vi "集成干预.vi"(11 "数据标记表":string(combo)="N") -> ()   [LabVIEW 2016, in "斯坦道多参数.lvlib"]
panel:
  out "运行状态":u16(ring) items=["空闲", "水样测试", "标样核查"]
  out "多参数运行日志":string
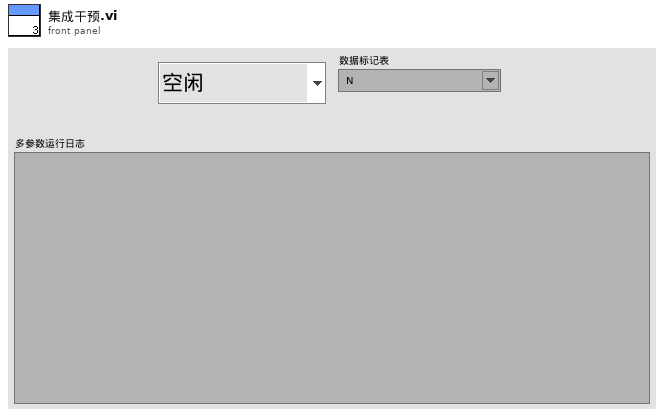
[diagram p1: front panel]
types:
  T1 = typedef "集成多参数单参数字段定义.ctl" = cluster{"时间":timestamp, "测量模式":string, "数据类型":string, "检测值":sgl, "单位":string, "数据标识":string, "信号值":sgl, "标样参考值":sgl, "因子编码":string, "探头温度":sgl, "LastTime":timestamp}
  T2 = cluster{"水温":bool, "pH":bool, "DO":bool, "DOper":bool, "电导率":bool, "ORP":bool, "浊度":bool, "叶绿素a":bool, "藻密度":bool, "COD":bool, "DO2":bool, "DOper":bool, "氯化物":bool, "氨氮":bool, "水中油":bool, "悬浮物":bool, "余氯":bool}
  T3 = cluster{"ph":bool, "DO":bool, "Cond":bool, "Turb":bool, "叶绿素a":bool, "藻密度":bool, "ORP":bool, "cod":bool, "DO2":bool, "氯化物":bool, "氨氮":bool, "水中油":bool, "悬浮物":bool, "余氯":bool}
  T4 = cluster{"温度测量值":sgl, "测量值":sgl, "温度偏移修正值":sgl, "信号值":sgl, "数据标识":string}
  T5 = cluster{"温度测量值":sgl, "DO%":sgl, "DOmg/L":sgl, "温度偏移修正值":sgl, "数据标识mg/L":string, "数据标识%":string}
  T6 = cluster{"CH":u16, "监测值":dbl, "信号值":sgl, "数据标识":string}
  T7 = cluster{"水样数据时间":timestamp, "水温":dbl, "pH":dbl, "DO":dbl, "DOper":dbl, "电导率":dbl, "ORP":dbl, "浊度":dbl, "叶绿素a":dbl, "藻密度":dbl, "COD":dbl, "DO2":dbl, "DO2per":dbl, "氯化物":dbl, "氨氮":dbl, "水中油":dbl, "悬浮物":dbl, "余氯":dbl}
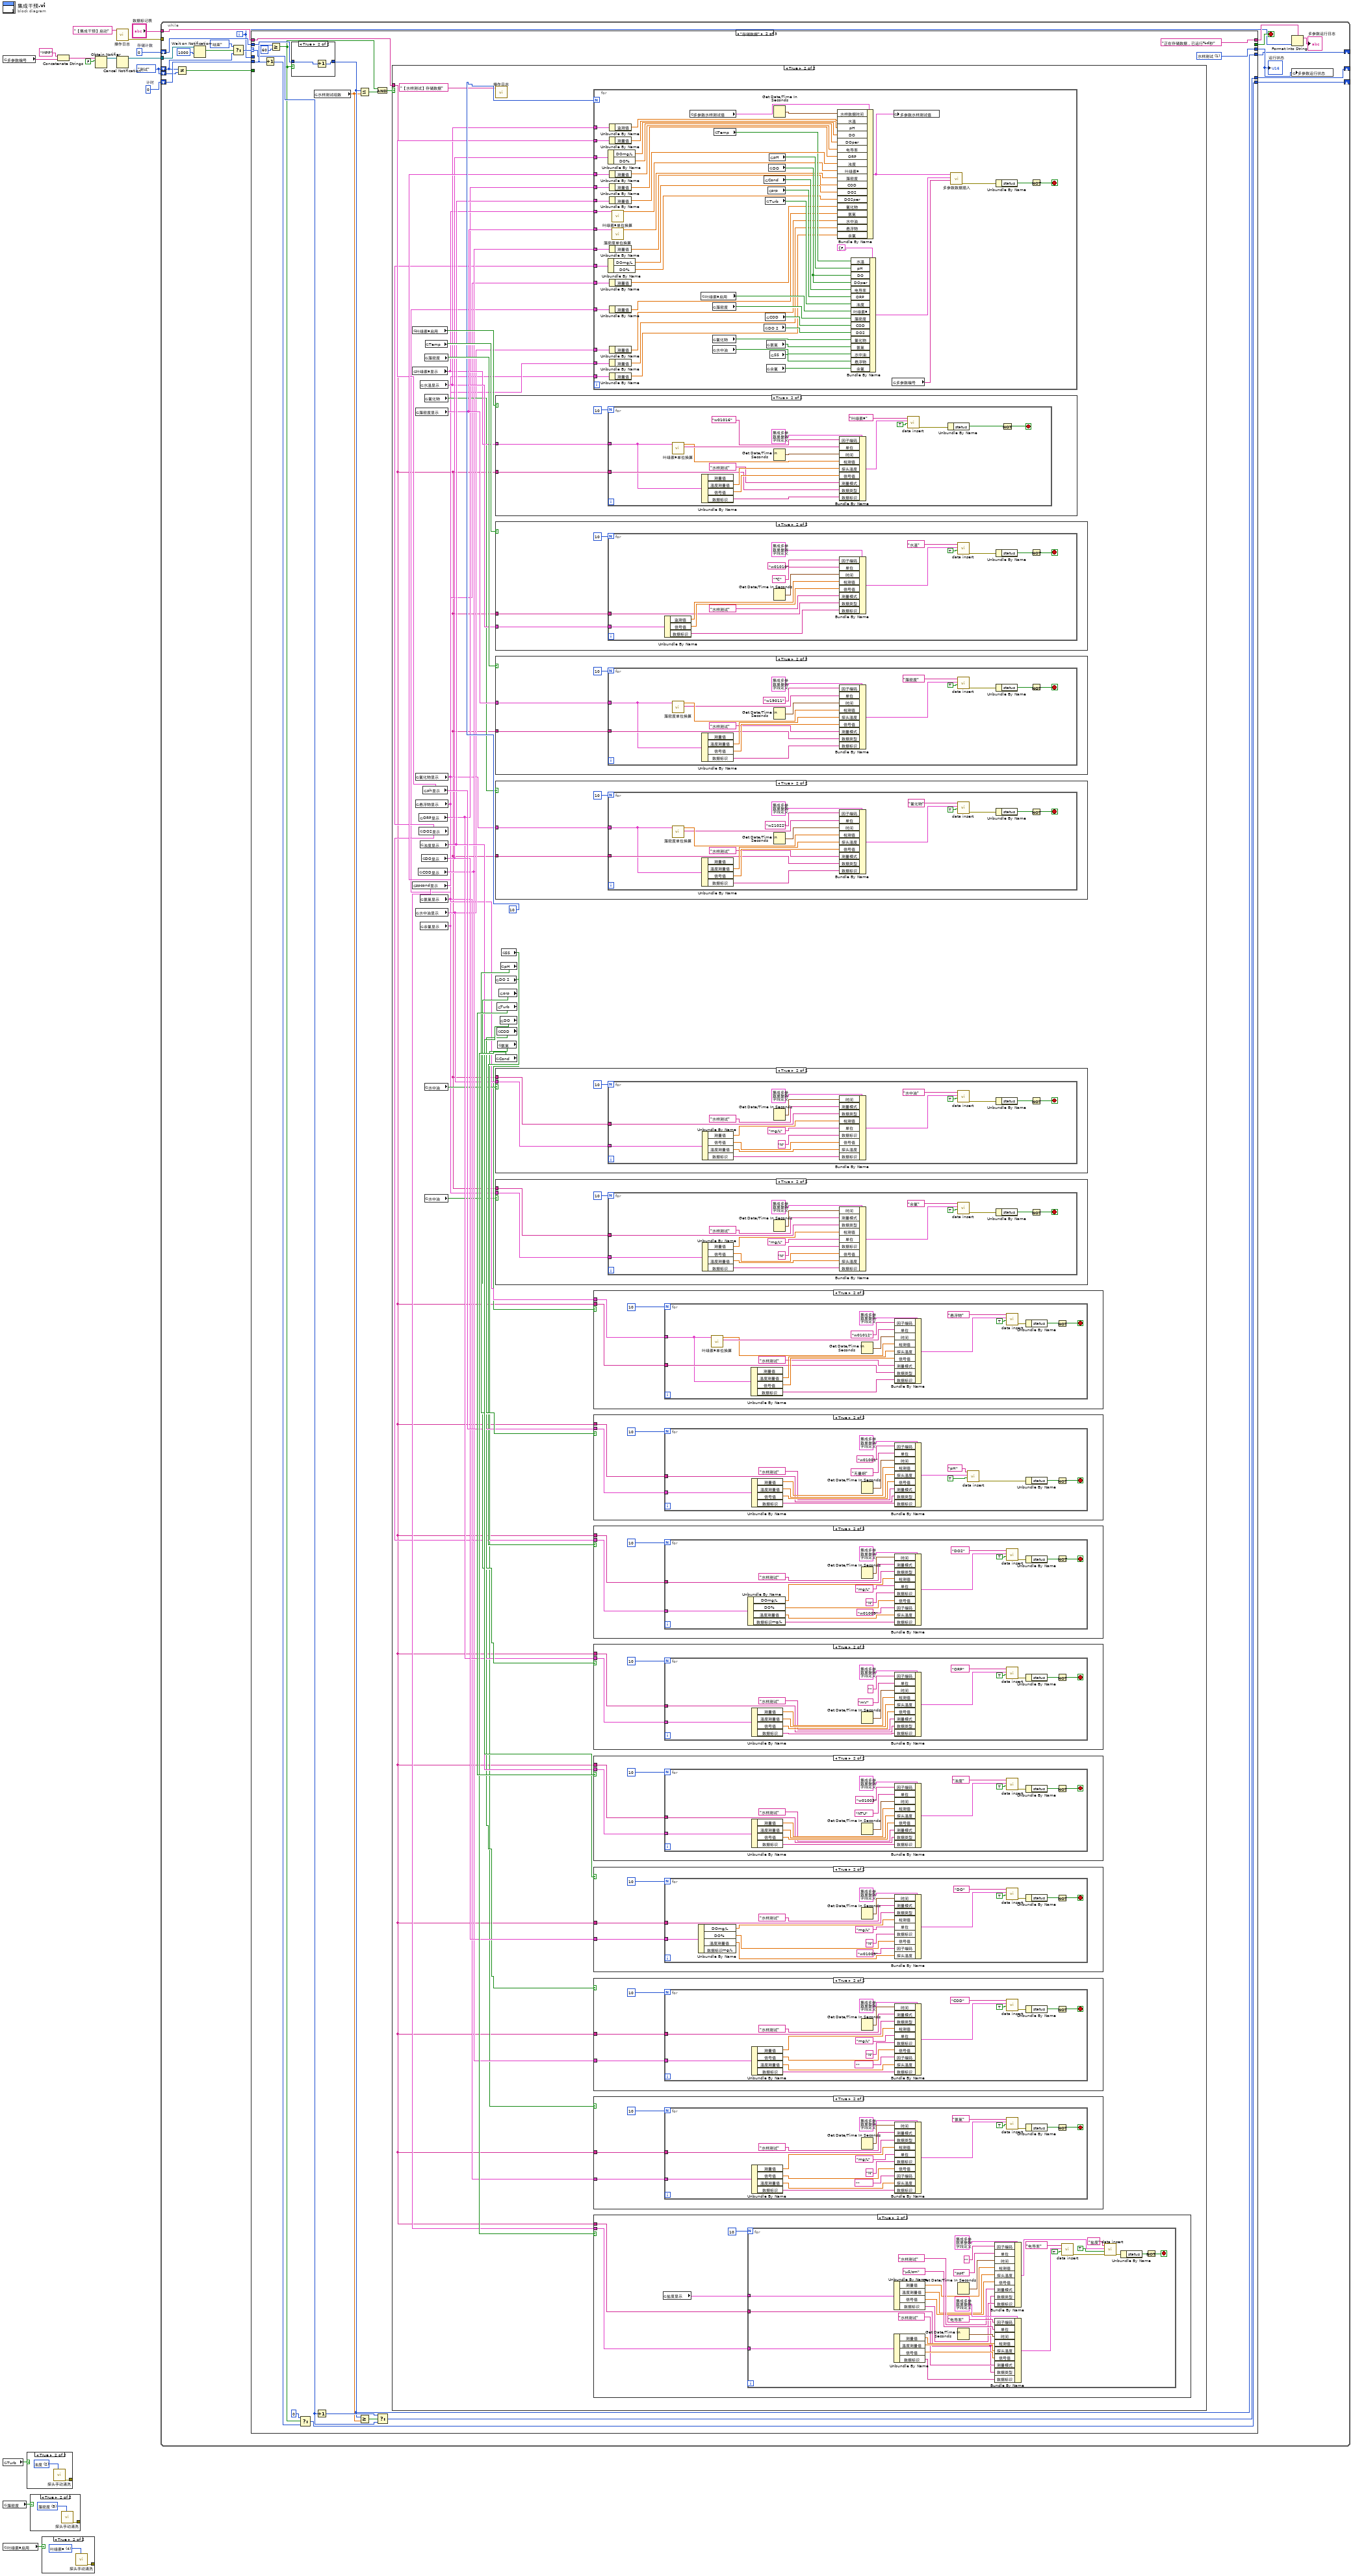
[diagram p0: block diagram]
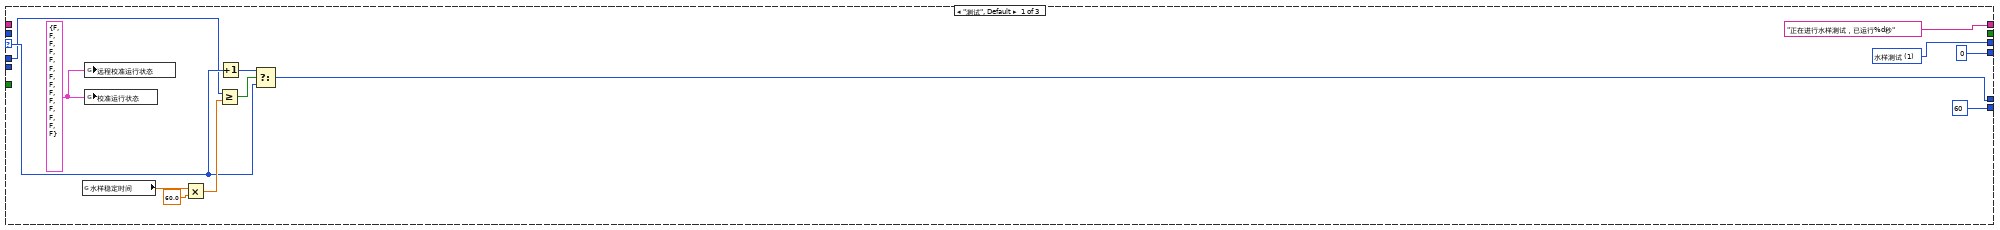
[diagram p5: hidden frame]
diagram:
  w7 = 0  # 存储计数
  w8 = 0  # 计时
  w3 = enum16{"测试", "存储数据", "结束"}."测试" ("枚举")
  n1 = global read "多参数全局变量.vi" "多参数编号"() -> (w9:string)
  n2 = global read "断电保存变量.vi" "Turb"() -> (w6:bool)
  n3 = global read "断电保存变量.vi" "藻密度"() -> (w4:bool)
  n4 = global read "断电保存变量.vi" "叶绿素a启用"() -> (w5:bool)
  n5 = case shown="True" w6 {
    tunnel: [_ w16] -> _
    frame False {
    }
    frame True {
      w17 = u16 2 items=["pH", "DO", "浊度", "电导率", "叶绿素a", "藻密度", "ORP", "DO2"] ("校准参数")
      n6 = call "探头手动清洗.vi"("校准参数"=w17) -> ("error out"=w16:errorcluster)  [unwired: 10 in]
    }
  }
  n7 = case shown="True" w4 {
    tunnel: [_ w18] -> _
    frame False {
    }
    frame True {
      w19 = u16 5 items=["pH", "DO", "浊度", "电导率", "叶绿素a", "藻密度", "ORP", "DO2"] ("校准参数")
      n8 = call "探头手动清洗.vi"("校准参数"=w19) -> ("error out"=w18:errorcluster)  [unwired: 10 in]
    }
  }
  n9 = case shown="True" w5 {
    tunnel: [_ w20] -> _
    frame False {
    }
    frame True {
      w21 = u16 4 items=["pH", "DO", "浊度", "电导率", "叶绿素a", "藻密度", "ORP", "DO2"] ("校准参数")
      n10 = call "探头手动清洗.vi"("校准参数"=w21) -> ("error out"=w20:errorcluster)  [unwired: 10 in]
    }
  }
  n11 = Concatenate Strings("MPP" ("名称（未命名）"), w9) -> (w10:string)
  n12 = Obtain Notifier(name (unnamed)=w10, notification data type=FALSE) -> (notifier out=w13:refnum<notifier>)  [unwired: 2 in, 2 out]
  n13 = call "操作日志.vi"("日志信息"="【集成干预】启动") -> ("error out"=w1:errorcluster)  [unwired: 10 in]
  n14 = Cancel Notification(0:w13) -> (8:w12:refnum<notifier>)  [unwired: 1 in, 2 out]
  n15 = while {
    shift-right: [w26] -> _
    shift-left: w3 -> [w24]
    tunnel: w12 -> [w37]
    tunnel: "数据标记表" -> [w32]
    shift-right: [w28] -> _
    shift-left: w8 -> [w30]
    shift-right: [w27] -> _
    shift-left: w7 -> [w29]
    shift-left: w3 -> [w23]
    tunnel: w1 -> [_]
    i -> [w25]
    stop <- w40 stop-if-true
    n16 = Not Equal?(x=w24, y=w23) -> (x != y?=w22:bool)
    n17 = Wait on Notification(notifier=w37, timeout in ms (-1)=1000 ("超时毫秒(-1)")) -> (notification=w35:bool)  [unwired: 2 in, 3 out]
    n18 = Select(t=enum16{"测试", "存储数据", "结束"}."结束" ("枚举"), s=w35, f=w24) -> (s? t:f=w33:enum16{"测试", "存储数据", "结束"})
    n19 = case shown="\"存储数据\"" w33 {
      selector: w33 -> [w47 w61 _]
      tunnel: [_ _ TRUE] -> w40
      tunnel: ["正在进行水样测试，已运行%d秒" ("格式字符串") "正在存储数据，已运行%d秒" ("格式字符串") "测试停止，累计运行%d秒" ("格式字符串")] -> w39
      tunnel: [w52 w66 w485] -> w31
      tunnel: w32 -> [_ w71 _]
      tunnel: w30 -> [_ w69 _]
      tunnel: w29 -> [_ w70 _]
      tunnel: [60 w54 0] -> w28
      tunnel: [0 w60 0] -> w27
      tunnel: [w45 w64 enum16{"测试", "存储数据", "结束"}."结束" ("枚举")] -> w26
      tunnel: w25 -> [w42 _ _]
      tunnel: w22 -> [_ _ w481]
      frame "测试", Default {
        w41 = T3 {"ph"=FALSE, "DO"=FALSE, "Cond"=FALSE, "Turb"=FALSE, "叶绿素a"=FALSE, "藻密度"=FALSE, "ORP"=FALSE, "cod"=FALSE, "DO2"=FALSE, "氯化物"=FALSE, "氨氮"=FALSE, "水中油"=FALSE, "悬浮物"=FALSE, "余氯"=FALSE} ("远程校准运行状态")
        w52 = u16 1 items=["空闲", "水样测试", "标样核查"] ("多参数运行状态")
        n20 = global read "断电保存变量.vi" "水样稳定时间"() -> (w51:dbl)
        n21 = global write "多参数全局变量.vi" "远程校准运行状态"(w41) -> ()
        n22 = global write "多参数全局变量.vi" "校准运行状态"(w41) -> ()
        n23 = Multiply(x=w51, y=60.0) -> (x*y=w49:dbl)
        n24 = Greater Or Equal?(x=w42, y=w49) -> (x >= y?=w48:bool)
        n25 = Increment(x=w47) -> (x+1=w46:enum16{"测试", "存储数据", "结束"})
        n26 = Select(t=w46, s=w48, f=w47) -> (s? t:f=w45:enum16{"测试", "存储数据", "结束"})
      }
      frame "存储数据" {
        w66 = u16 1 items=["空闲", "水样测试", "标样核查"] ("多参数运行状态")
        n27 = Increment(x=w69) -> (x+1=w56:i32)
        n28 = Greater Or Equal?(x=w69, y=60) -> (x >= y?=w57:bool)
        n29 = case shown="True" w57 {
          tunnel: w70 -> [w72 w74]
          tunnel: [w72 w73] -> w60
          frame False {
          }
          frame True {
            n30 = Increment(x=w74) -> (x+1=w73:i32)
          }
        }
        n31 = Select(t=0, s=w57, f=w56) -> (s? t:f=w54:i32)
        n32 = global read "断电保存变量.vi" "水样测试组数"() -> (w59:dbl)
        n33 = Increment(x=w61) -> (x+1=w62:enum16{"测试", "存储数据", "结束"})
        n34 = Less Or Equal?(x=w60, y=w59) -> (x <= y?=w65:bool)
        n35 = Greater Or Equal?(x=w60, y=w59) -> (x >= y?=w58:bool)
        n36 = And(x=w57, y=w65) -> (x .and. y?=w63:bool)
        n37 = Select(t=w62, s=w58, f=w61) -> (s? t:f=w64:enum16{"测试", "存储数据", "结束"})
        n38 = case shown="True" w63 {
          tunnel: w71 -> [_ w75]
          frame False {
          }
          frame True {
            n39 = global read "断电保存变量.vi" "叶绿素a启用"() -> (w107:bool)
            n40 = global read "多参数全局变量.vi" "叶绿素a显示"() -> (w92:T4)
            n41 = global read "多参数全局变量.vi" "spcond显示"() -> (w98:T4)
            n42 = global read "多参数全局变量.vi" "藻密度显示"() -> (w94:T4)
            n43 = global read "多参数全局变量.vi" "氯化物显示"() -> (w84:T4)
            n44 = global read "多参数全局变量.vi" "悬浮物显示"() -> (w79:T4)
            n45 = global read "多参数全局变量.vi" "水中油显示"() -> (w80:T4)
            n46 = global read "多参数全局变量.vi" "COD显示"() -> (w89:T4)
            n47 = global read "多参数全局变量.vi" "ORP显示"() -> (w91:T4)
            n48 = global read "多参数全局变量.vi" "DO2显示"() -> (w86:T5)
            n49 = global read "多参数全局变量.vi" "水温显示"() -> (w93:T6)
            n50 = global read "多参数全局变量.vi" "浊度显示"() -> (w96:T4)
            n51 = global read "多参数全局变量.vi" "氨氮显示"() -> (w82:T4)
            n52 = global read "多参数全局变量.vi" "余氯显示"() -> (w76:T4)
            n53 = global read "多参数全局变量.vi" "DO显示"() -> (w95:T5)
            n54 = global read "多参数全局变量.vi" "ph显示"() -> (w97:T4)
            n55 = global read "断电保存变量.vi" "藻密度"() -> (w101:bool)
            n56 = global read "断电保存变量.vi" "氯化物"() -> (w85:bool)
            n57 = global read "断电保存变量.vi" "水中油"() -> (w81:bool)
            n58 = global read "断电保存变量.vi" "水中油"() -> (w77:bool)
            n59 = global read "断电保存变量.vi" "Temp"() -> (w102:bool)
            n60 = call "操作日志.vi"("日志信息"="【水样测试】存储数据") -> ()  [unwired: 10 in, 1 out]
            n61 = case shown="True" w107 {
              tunnel: w75 -> [_ w349]
              tunnel: w92 -> [_ w347]
              frame False {
              }
              frame True {
                n62 = for {
                  N: 10 -> [_]
                  tunnel: w349 -> [w356]
                  tunnel: w347 -> [w353]
                  stop <- w360 stop-if-true
                  n63 = call "叶绿素a单位换算.vi"("叶绿素a显示"=w353) -> ("检测值1.单位"=w352:string, "测量值"=w351:sgl)  [unwired: 8 in, 1 out]
                  n64 = Unbundle By Name(w353) -> ("温度测量值"=w366:sgl, "信号值"=w359:sgl, "数据标识"=w355:string)  [unwired: 1 out]
                  n65 = Get Date/Time In Seconds() -> (seconds since 1Jan1904=w358:timestamp)
                  n66 = Bundle By Name(cluster=T1 {"时间"=timestamp(0 s since 1904-01-01), "测量模式"="水样测试", "数据类型"="N", "检测值"=0.0, "单位"="mg/L", "数据标识"="N", "信号值"=0.0, "标样参考值"=0.0, "因子编码"="", "探头温度"=0.0, "LastTime"=timestamp(0 s since 1904-01-01)} ("data"), "因子编码"="w01016", "单位"=w352, "时间"=w358, "检测值"=w351, "探头温度"=w366, "信号值"=w359, "测量模式"="水样测试", "数据类型"=w356, "数据标识"=w355) -> (w364:T1)
                  n67 = call "data insert.vi"("集成干预"=TRUE, "data"=w364, "table in"="叶绿素a" ("table输入")) -> ("error out"=w362:errorcluster)  [unwired: 8 in]
                  n68 = Unbundle By Name(w362) -> ("status"=w361:bool)
                  n69 = Not(x=w361) -> (.not. x?=w360:bool)
                }
              }
            }
            n70 = case shown="True" w102 {
              tunnel: w75 -> [_ w464]
              tunnel: w93 -> [_ w462]
              frame False {
              }
              frame True {
                n71 = for {
                  N: 10 -> [_]
                  tunnel: w464 -> [w469]
                  tunnel: w462 -> [w468]
                  stop <- w473 stop-if-true
                  n72 = Unbundle By Name(w468) -> ("监测值"=w476:dbl, "信号值"=w471:sgl, "数据标识"=w467:string)
                  n73 = Get Date/Time In Seconds() -> (seconds since 1Jan1904=w472:timestamp)
                  n74 = Bundle By Name(cluster=T1 {"时间"=timestamp(0 s since 1904-01-01), "测量模式"="水样测试", "数据类型"="N", "检测值"=0.0, "单位"="mg/L", "数据标识"="N", "信号值"=0.0, "标样参考值"=0.0, "因子编码"="", "探头温度"=0.0, "LastTime"=timestamp(0 s since 1904-01-01)} ("data"), "因子编码"="w01010", "单位"="℃", "时间"=w472, "检测值"=w476, "信号值"=w471, "测量模式"="水样测试", "数据类型"=w469, "数据标识"=w467) -> (w479:T1)
                  n75 = call "data insert.vi"("集成干预"=TRUE, "data"=w479, "table in"="水温" ("table输入")) -> ("error out"=w475:errorcluster)  [unwired: 8 in]
                  n76 = Unbundle By Name(w475) -> ("status"=w474:bool)
                  n77 = Not(x=w474) -> (.not. x?=w473:bool)
                }
              }
            }
            n78 = case shown="True" w101 {
              tunnel: w75 -> [_ w329]
              tunnel: w94 -> [_ w327]
              frame False {
              }
              frame True {
                n79 = for {
                  N: 10 -> [_]
                  tunnel: w329 -> [w337]
                  tunnel: w327 -> [w333]
                  stop <- w338 stop-if-true
                  n80 = call "藻密度单位换算.vi"("藻密度显示"=w333) -> ("检测值1.单位"=w331:string, "测量值"=w332:sgl)  [unwired: 8 in, 1 out]
                  n81 = Unbundle By Name(w333) -> ("温度测量值"=w346:sgl, "信号值"=w339:sgl, "数据标识"=w335:string)  [unwired: 1 out]
                  n82 = Get Date/Time In Seconds() -> (seconds since 1Jan1904=w340:timestamp)
                  n83 = Bundle By Name(cluster=T1 {"时间"=timestamp(0 s since 1904-01-01), "测量模式"="水样测试", "数据类型"="N", "检测值"=0.0, "单位"="mg/L", "数据标识"="N", "信号值"=0.0, "标样参考值"=0.0, "因子编码"="", "探头温度"=0.0, "LastTime"=timestamp(0 s since 1904-01-01)} ("data"), "因子编码"="w19011", "单位"=w331, "时间"=w340, "检测值"=w332, "探头温度"=w346, "信号值"=w339, "测量模式"="水样测试", "数据类型"=w337, "数据标识"=w335) -> (w341:T1)
                  n84 = call "data insert.vi"("集成干预"=TRUE, "data"=w341, "table in"="藻密度" ("table输入")) -> ("error out"=w343:errorcluster)  [unwired: 8 in]
                  n85 = Unbundle By Name(w343) -> ("status"=w342:bool)
                  n86 = Not(x=w342) -> (.not. x?=w338:bool)
                }
              }
            }
            n87 = case shown="True" w85 {
              tunnel: w75 -> [_ w191]
              tunnel: w84 -> [_ w189]
              frame False {
              }
              frame True {
                n88 = for {
                  N: 10 -> [_]
                  tunnel: w191 -> [w201]
                  tunnel: w189 -> [w197]
                  stop <- w202 stop-if-true
                  n89 = call "藻密度单位换算.vi"("藻密度显示"=w197) -> ("检测值1.单位"=w195:string, "测量值"=w196:sgl)  [unwired: 8 in, 1 out]
                  n90 = Unbundle By Name(w197) -> ("温度测量值"=w208:sgl, "信号值"=w203:sgl, "数据标识"=w199:string)  [unwired: 1 out]
                  n91 = Get Date/Time In Seconds() -> (seconds since 1Jan1904=w204:timestamp)
                  n92 = Bundle By Name(cluster=T1 {"时间"=timestamp(0 s since 1904-01-01), "测量模式"="水样测试", "数据类型"="N", "检测值"=0.0, "单位"="mg/L", "数据标识"="N", "信号值"=0.0, "标样参考值"=0.0, "因子编码"="", "探头温度"=0.0, "LastTime"=timestamp(0 s since 1904-01-01)} ("data"), "因子编码"="w21022", "单位"=w195, "时间"=w204, "检测值"=w196, "探头温度"=w208, "信号值"=w203, "测量模式"="水样测试", "数据类型"=w201, "数据标识"=w199) -> (w205:T1)
                  n93 = call "data insert.vi"("集成干预"=TRUE, "data"=w205, "table in"="氯化物") -> ("error out"=w207:errorcluster)  [unwired: 8 in]
                  n94 = Unbundle By Name(w207) -> ("status"=w206:bool)
                  n95 = Not(x=w206) -> (.not. x?=w202:bool)
                }
              }
            }
            n96 = global read "断电保存变量.vi" "DO 2"() -> (w87:bool)
            n97 = global read "断电保存变量.vi" "Cond"() -> (w105:bool)
            n98 = case shown="True" w81 {
              tunnel: w75 -> [_ w150]
              tunnel: w80 -> [_ w148]
              frame False {
              }
              frame True {
                n99 = for {
                  N: 10 -> [_]
                  tunnel: w150 -> [w164]
                  tunnel: w148 -> [w157]
                  stop <- w167 stop-if-true
                  n100 = Unbundle By Name(w157) -> ("测量值"=w156:sgl, "信号值"=w155:sgl, "温度测量值"=w154:sgl, "数据标识"=w153:string)
                  n101 = Get Date/Time In Seconds() -> (seconds since 1Jan1904=w166:timestamp)
                  n102 = Bundle By Name(cluster=T1 {"时间"=timestamp(0 s since 1904-01-01), "测量模式"="水样测试", "数据类型"="N", "检测值"=0.0, "单位"="mg/L", "数据标识"="N", "信号值"=0.0, "标样参考值"=0.0, "因子编码"="", "探头温度"=0.0, "LastTime"=timestamp(0 s since 1904-01-01)} ("data"), "时间"=w166, "测量模式"="水样测试", "数据类型"=w164, "检测值"=w156, "单位"="mg/L", "数据标识"="N" ("水样数据标识"), "信号值"=w155, "探头温度"=w154, "数据标识"=w153) -> (w159:T1)
                  n103 = call "data insert.vi"("集成干预"=TRUE, "data"=w159, "table in"="水中油") -> ("error out"=w160:errorcluster)  [unwired: 8 in]
                  n104 = Unbundle By Name(w160) -> ("status"=w161:bool)
                  n105 = Not(x=w161) -> (.not. x?=w167:bool)
                }
              }
            }
            n106 = case shown="True" w77 {
              tunnel: w75 -> [_ w110]
              tunnel: w76 -> [_ w108]
              frame False {
              }
              frame True {
                n107 = for {
                  N: 10 -> [_]
                  tunnel: w110 -> [w124]
                  tunnel: w108 -> [w117]
                  stop <- w127 stop-if-true
                  n108 = Unbundle By Name(w117) -> ("测量值"=w116:sgl, "信号值"=w115:sgl, "温度测量值"=w114:sgl, "数据标识"=w113:string)
                  n109 = Get Date/Time In Seconds() -> (seconds since 1Jan1904=w126:timestamp)
                  n110 = Bundle By Name(cluster=T1 {"时间"=timestamp(0 s since 1904-01-01), "测量模式"="水样测试", "数据类型"="N", "检测值"=0.0, "单位"="mg/L", "数据标识"="N", "信号值"=0.0, "标样参考值"=0.0, "因子编码"="", "探头温度"=0.0, "LastTime"=timestamp(0 s since 1904-01-01)} ("data"), "时间"=w126, "测量模式"="水样测试", "数据类型"=w124, "检测值"=w116, "单位"="mg/L", "数据标识"="N" ("水样数据标识"), "信号值"=w115, "探头温度"=w114, "数据标识"=w113) -> (w119:T1)
                  n111 = call "data insert.vi"("集成干预"=TRUE, "data"=w119, "table in"="余氯") -> ("error out"=w120:errorcluster)  [unwired: 8 in]
                  n112 = Unbundle By Name(w120) -> ("status"=w121:bool)
                  n113 = Not(x=w121) -> (.not. x?=w127:bool)
                }
              }
            }
            n114 = global read "断电保存变量.vi" "Turb"() -> (w106:bool)
            n115 = global read "断电保存变量.vi" "COD"() -> (w88:bool)
            n116 = global read "断电保存变量.vi" "氨氮"() -> (w83:bool)
            n117 = global read "断电保存变量.vi" "orp"() -> (w100:bool)
            n118 = global read "断电保存变量.vi" "DO"() -> (w104:bool)
            n119 = global read "断电保存变量.vi" "pH"() -> (w103:bool)
            n120 = global read "断电保存变量.vi" "SS"() -> (w78:bool)
            n121 = for {
              N: 10 -> [_]
              tunnel: w93 -> [w286]
              tunnel: w97 -> [w285]
              tunnel: w95 -> [w284]
              tunnel: w98 -> [w283]
              tunnel: w91 -> [w282]
              tunnel: w96 -> [w281]
              tunnel: w92 -> [w271]
              tunnel: w94 -> [w273]
              tunnel: w89 -> [w279]
              tunnel: w86 -> [w276]
              tunnel: w84 -> [w267]
              tunnel: w82 -> [w265]
              tunnel: w80 -> [w260]
              tunnel: w79 -> [w254]
              tunnel: w76 -> [w252]
              stop <- w288 stop-if-true
              n122 = Unbundle By Name(w284) -> ("DOmg/L"=w303:sgl, "DO%"=w302:sgl)
              n123 = Unbundle By Name(w276) -> ("DOmg/L"=w275:sgl, "DO%"=w274:sgl)
              n124 = Unbundle By Name(w286) -> ("监测值"=w305:dbl)
              n125 = Unbundle By Name(w285) -> ("测量值"=w304:sgl)
              n126 = Unbundle By Name(w283) -> ("测量值"=w301:sgl)
              n127 = Unbundle By Name(w282) -> ("测量值"=w300:sgl)
              n128 = Unbundle By Name(w281) -> ("测量值"=w299:sgl)
              n129 = Unbundle By Name(w279) -> ("测量值"=w278:sgl)
              n130 = Unbundle By Name(w267) -> ("测量值"=w266:sgl)
              n131 = Unbundle By Name(w265) -> ("测量值"=w264:sgl)
              n132 = Unbundle By Name(w260) -> ("测量值"=w259:sgl)
              n133 = Unbundle By Name(w254) -> ("测量值"=w255:sgl)
              n134 = Unbundle By Name(w252) -> ("测量值"=w251:sgl)
              n135 = call "叶绿素a单位换算.vi"("叶绿素a显示"=w271) -> ("测量值"=w270:sgl)  [unwired: 8 in, 2 out]
              n136 = call "藻密度单位换算.vi"("藻密度显示"=w273) -> ("测量值"=w272:sgl)  [unwired: 8 in, 2 out]
              n137 = global read "多参数全局变量.vi" "多参数水样测试值"() -> (w262:T7)
              n138 = global read "断电保存变量.vi" "叶绿素a启用"() -> (w292:bool)
              n139 = global read "断电保存变量.vi" "藻密度"() -> (w295:bool)
              n140 = global read "断电保存变量.vi" "氯化物"() -> (w268:bool)
              n141 = global read "断电保存变量.vi" "水中油"() -> (w261:bool)
              n142 = global read "断电保存变量.vi" "Temp"() -> (w294:bool)
              n143 = global read "断电保存变量.vi" "Cond"() -> (w297:bool)
              n144 = global read "断电保存变量.vi" "DO 2"() -> (w277:bool)
              n145 = global read "断电保存变量.vi" "Turb"() -> (w296:bool)
              n146 = global read "断电保存变量.vi" "COD"() -> (w280:bool)
              n147 = global read "断电保存变量.vi" "氨氮"() -> (w263:bool)
              n148 = global read "断电保存变量.vi" "余氯"() -> (w253:bool)
              n149 = global read "断电保存变量.vi" "orp"() -> (w293:bool)
              n150 = global read "断电保存变量.vi" "DO"() -> (w291:bool)
              n151 = global read "断电保存变量.vi" "pH"() -> (w298:bool)
              n152 = global read "断电保存变量.vi" "SS"() -> (w258:bool)
              n153 = Get Date/Time In Seconds() -> (seconds since 1Jan1904=w306:timestamp)
              n154 = Bundle By Name(cluster=w262, "水样数据时间"=w306, "水温"=w305, "pH"=w304, "DO"=w303, "DOper"=w302, "电导率"=w301, "ORP"=w300, "浊度"=w299, "叶绿素a"=w270, "藻密度"=w272, "COD"=w278, "DO2"=w275, "DO2per"=w274, "氯化物"=w266, "氨氮"=w264, "水中油"=w259, "悬浮物"=w255, "余氯"=w251) -> (w269:T7)
              n155 = Bundle By Name(cluster=T2 {"水温"=FALSE, "pH"=FALSE, "DO"=FALSE, "DOper"=FALSE, "电导率"=FALSE, "ORP"=FALSE, "浊度"=FALSE, "叶绿素a"=FALSE, "藻密度"=FALSE, "COD"=FALSE, "DO2"=FALSE, "DOper"=FALSE, "氯化物"=FALSE, "氨氮"=FALSE, "水中油"=FALSE, "悬浮物"=FALSE, "余氯"=FALSE} ("columns enable"), "水温"=w294, "pH"=w298, "DO"=w291, "DOper"=w291, "电导率"=w297, "ORP"=w293, "浊度"=w296, "叶绿素a"=w292, "藻密度"=w295, "COD"=w280, "DO2"=w277, "氯化物"=w268, "氨氮"=w263, "水中油"=w261, "悬浮物"=w258, "余氯"=w253) -> (w256:T2)
              n156 = global read "多参数全局变量.vi" "多参数编号"() -> (w287:string)
              n157 = global write "多参数全局变量.vi" "多参数水样测试值"(w269) -> ()
              n158 = call "多参数数据插入.vi"("编号"=w287, "columns enable"=w256, "data in"=w269) -> ("error out"=w290:errorcluster)  [unwired: 8 in]
              n159 = Unbundle By Name(w290) -> ("status"=w289:bool)
              n160 = Not(x=w289) -> (.not. x?=w288:bool)
            }
            n161 = case shown="True" w78 {
              tunnel: w75 -> [_ w130]
              tunnel: w79 -> [_ w128]
              frame False {
              }
              frame True {
                n162 = for {
                  N: 10 -> [_]
                  tunnel: w130 -> [w137]
                  tunnel: w128 -> [w134]
                  stop <- w141 stop-if-true
                  n163 = call "叶绿素a单位换算.vi"("叶绿素a显示"=w134) -> ("检测值1.单位"=w133:string, "测量值"=w132:sgl)  [unwired: 8 in, 1 out]
                  n164 = Unbundle By Name(w134) -> ("温度测量值"=w147:sgl, "信号值"=w140:sgl, "数据标识"=w136:string)  [unwired: 1 out]
                  n165 = Get Date/Time In Seconds() -> (seconds since 1Jan1904=w139:timestamp)
                  n166 = Bundle By Name(cluster=T1 {"时间"=timestamp(0 s since 1904-01-01), "测量模式"="水样测试", "数据类型"="N", "检测值"=0.0, "单位"="mg/L", "数据标识"="N", "信号值"=0.0, "标样参考值"=0.0, "因子编码"="", "探头温度"=0.0, "LastTime"=timestamp(0 s since 1904-01-01)} ("data"), "因子编码"="w01012", "单位"=w133, "时间"=w139, "检测值"=w132, "探头温度"=w147, "信号值"=w140, "测量模式"="水样测试", "数据类型"=w137, "数据标识"=w136) -> (w145:T1)
                  n167 = call "data insert.vi"("集成干预"=TRUE, "data"=w145, "table in"="悬浮物" ("table输入")) -> ("error out"=w143:errorcluster)  [unwired: 8 in]
                  n168 = Unbundle By Name(w143) -> ("status"=w142:bool)
                  n169 = Not(x=w142) -> (.not. x?=w141:bool)
                }
              }
            }
            n170 = case shown="True" w103 {
              tunnel: w75 -> [_ w444]
              tunnel: w97 -> [_ w442]
              frame False {
              }
              frame True {
                n171 = for {
                  N: 10 -> [_]
                  tunnel: w444 -> [w449]
                  tunnel: w442 -> [w448]
                  stop <- w453 stop-if-true
                  n172 = Unbundle By Name(w448) -> ("测量值"=w457:sgl, "温度测量值"=w456:sgl, "信号值"=w451:sgl, "数据标识"=w447:string)
                  n173 = Get Date/Time In Seconds() -> (seconds since 1Jan1904=w452:timestamp)
                  n174 = Bundle By Name(cluster=T1 {"时间"=timestamp(0 s since 1904-01-01), "测量模式"="水样测试", "数据类型"="N", "检测值"=0.0, "单位"="mg/L", "数据标识"="N", "信号值"=0.0, "标样参考值"=0.0, "因子编码"="", "探头温度"=0.0, "LastTime"=timestamp(0 s since 1904-01-01)} ("data"), "因子编码"="w01001", "单位"="无量纲", "时间"=w452, "检测值"=w457, "探头温度"=w456, "信号值"=w451, "测量模式"="水样测试", "数据类型"=w449, "数据标识"=w447) -> (w461:T1)
                  n175 = call "data insert.vi"("集成干预"=TRUE, "data"=w461, "table in"="pH" ("table输入")) -> ("error out"=w455:errorcluster)  [unwired: 8 in]
                  n176 = Unbundle By Name(w455) -> ("status"=w454:bool)
                  n177 = Not(x=w454) -> (.not. x?=w453:bool)
                }
              }
            }
            n178 = case shown="True" w87 {
              tunnel: w75 -> [_ w211]
              tunnel: w86 -> [_ w209]
              frame False {
              }
              frame True {
                n179 = for {
                  N: 10 -> [_]
                  tunnel: w211 -> [w226]
                  tunnel: w209 -> [w216]
                  stop <- w229 stop-if-true
                  n180 = Unbundle By Name(w216) -> ("DOmg/L"=w225:sgl, "DO%"=w218:sgl, "温度测量值"=w219:sgl, "数据标识mg/L"=w215:string)
                  n181 = Get Date/Time In Seconds() -> (seconds since 1Jan1904=w228:timestamp)
                  n182 = Bundle By Name(cluster=T1 {"时间"=timestamp(0 s since 1904-01-01), "测量模式"="水样测试", "数据类型"="N", "检测值"=0.0, "单位"="mg/L", "数据标识"="N", "信号值"=0.0, "标样参考值"=0.0, "因子编码"="", "探头温度"=0.0, "LastTime"=timestamp(0 s since 1904-01-01)} ("data"), "时间"=w228, "测量模式"="水样测试", "数据类型"=w226, "检测值"=w225, "单位"="mg/L", "数据标识"="N" ("水样数据标识"), "信号值"=w218, "因子编码"="w01009", "探头温度"=w219, "数据标识"=w215) -> (w217:T1)
                  n183 = call "data insert.vi"("集成干预"=TRUE, "data"=w217, "table in"="DO2") -> ("error out"=w221:errorcluster)  [unwired: 8 in]
                  n184 = Unbundle By Name(w221) -> ("status"=w222:bool)
                  n185 = Not(x=w222) -> (.not. x?=w229:bool)
                }
              }
            }
            n186 = case shown="True" w100 {
              tunnel: w75 -> [_ w309]
              tunnel: w91 -> [_ w307]
              frame False {
              }
              frame True {
                n187 = for {
                  N: 10 -> [_]
                  tunnel: w309 -> [w316]
                  tunnel: w307 -> [w314]
                  stop <- w319 stop-if-true
                  n188 = Unbundle By Name(w314) -> ("测量值"=w326:sgl, "温度测量值"=w324:sgl, "信号值"=w317:sgl, "数据标识"=w313:string)
                  n189 = Get Date/Time In Seconds() -> (seconds since 1Jan1904=w318:timestamp)
                  n190 = Bundle By Name(cluster=T1 {"时间"=timestamp(0 s since 1904-01-01), "测量模式"="水样测试", "数据类型"="N", "检测值"=0.0, "单位"="mg/L", "数据标识"="N", "信号值"=0.0, "标样参考值"=0.0, "因子编码"="", "探头温度"=0.0, "LastTime"=timestamp(0 s since 1904-01-01)} ("data"), "因子编码"="", "单位"="mV", "时间"=w318, "检测值"=w326, "探头温度"=w324, "信号值"=w317, "测量模式"="水样测试", "数据类型"=w316, "数据标识"=w313) -> (w311:T1)
                  n191 = call "data insert.vi"("集成干预"=TRUE, "data"=w311, "table in"="ORP" ("table输入")) -> ("error out"=w322:errorcluster)  [unwired: 8 in]
                  n192 = Unbundle By Name(w322) -> ("status"=w321:bool)
                  n193 = Not(x=w321) -> (.not. x?=w319:bool)
                }
              }
            }
            n194 = case shown="True" w106 {
              tunnel: w75 -> [_ w369]
              tunnel: w96 -> [_ w367]
              frame False {
              }
              frame True {
                n195 = for {
                  N: 10 -> [_]
                  tunnel: w369 -> [w374]
                  tunnel: w367 -> [w373]
                  stop <- w378 stop-if-true
                  n196 = Unbundle By Name(w373) -> ("测量值"=w382:sgl, "温度测量值"=w381:sgl, "信号值"=w376:sgl, "数据标识"=w372:string)
                  n197 = Get Date/Time In Seconds() -> (seconds since 1Jan1904=w377:timestamp)
                  n198 = Bundle By Name(cluster=T1 {"时间"=timestamp(0 s since 1904-01-01), "测量模式"="水样测试", "数据类型"="N", "检测值"=0.0, "单位"="mg/L", "数据标识"="N", "信号值"=0.0, "标样参考值"=0.0, "因子编码"="", "探头温度"=0.0, "LastTime"=timestamp(0 s since 1904-01-01)} ("data"), "因子编码"="w01003", "单位"="NTU", "时间"=w377, "检测值"=w382, "探头温度"=w381, "信号值"=w376, "测量模式"="水样测试", "数据类型"=w374, "数据标识"=w372) -> (w385:T1)
                  n199 = call "data insert.vi"("集成干预"=TRUE, "data"=w385, "table in"="浊度" ("table输入")) -> ("error out"=w380:errorcluster)  [unwired: 8 in]
                  n200 = Unbundle By Name(w380) -> ("status"=w379:bool)
                  n201 = Not(x=w379) -> (.not. x?=w378:bool)
                }
              }
            }
            n202 = case shown="True" w104 {
              tunnel: w75 -> [_ w424]
              tunnel: w95 -> [_ w422]
              frame False {
              }
              frame True {
                n203 = for {
                  N: 10 -> [_]
                  tunnel: w424 -> [w437]
                  tunnel: w422 -> [w428]
                  stop <- w441 stop-if-true
                  n204 = Unbundle By Name(w428) -> ("DOmg/L"=w436:sgl, "DO%"=w430:sgl, "温度测量值"=w431:sgl)  [unwired: 1 out]
                  n205 = Get Date/Time In Seconds() -> (seconds since 1Jan1904=w439:timestamp)
                  n206 = Bundle By Name(cluster=T1 {"时间"=timestamp(0 s since 1904-01-01), "测量模式"="水样测试", "数据类型"="N", "检测值"=0.0, "单位"="mg/L", "数据标识"="N", "信号值"=0.0, "标样参考值"=0.0, "因子编码"="", "探头温度"=0.0, "LastTime"=timestamp(0 s since 1904-01-01)} ("data"), "时间"=w439, "测量模式"="水样测试", "数据类型"=w437, "检测值"=w436, "单位"="mg/L", "数据标识"="N", "信号值"=w430, "因子编码"="w01009", "探头温度"=w431) -> (w429:T1)
                  n207 = call "data insert.vi"("集成干预"=TRUE, "data"=w429, "table in"="DO") -> ("error out"=w433:errorcluster)  [unwired: 8 in]
                  n208 = Unbundle By Name(w433) -> ("status"=w434:bool)
                  n209 = Not(x=w434) -> (.not. x?=w441:bool)
                }
              }
            }
            n210 = case shown="True" w88 {
              tunnel: w75 -> [_ w232]
              tunnel: w89 -> [_ w230]
              frame False {
              }
              frame True {
                n211 = for {
                  N: 10 -> [_]
                  tunnel: w232 -> [w246]
                  tunnel: w230 -> [w236]
                  stop <- w250 stop-if-true
                  n212 = Unbundle By Name(w236) -> ("测量值"=w245:sgl, "信号值"=w238:sgl, "温度测量值"=w239:sgl, "数据标识"=w235:string)
                  n213 = Get Date/Time In Seconds() -> (seconds since 1Jan1904=w248:timestamp)
                  n214 = Bundle By Name(cluster=T1 {"时间"=timestamp(0 s since 1904-01-01), "测量模式"="水样测试", "数据类型"="N", "检测值"=0.0, "单位"="mg/L", "数据标识"="N", "信号值"=0.0, "标样参考值"=0.0, "因子编码"="", "探头温度"=0.0, "LastTime"=timestamp(0 s since 1904-01-01)} ("data"), "时间"=w248, "测量模式"="水样测试", "数据类型"=w246, "检测值"=w245, "单位"="mg/L", "数据标识"="N" ("水样数据标识"), "信号值"=w238, "因子编码"="", "探头温度"=w239, "数据标识"=w235) -> (w237:T1)
                  n215 = call "data insert.vi"("集成干预"=TRUE, "data"=w237, "table in"="COD") -> ("error out"=w241:errorcluster)  [unwired: 8 in]
                  n216 = Unbundle By Name(w241) -> ("status"=w242:bool)
                  n217 = Not(x=w242) -> (.not. x?=w250:bool)
                }
              }
            }
            n218 = case shown="True" w83 {
              tunnel: w75 -> [_ w170]
              tunnel: w82 -> [_ w168]
              frame False {
              }
              frame True {
                n219 = for {
                  N: 10 -> [_]
                  tunnel: w170 -> [w184]
                  tunnel: w168 -> [w176]
                  stop <- w188 stop-if-true
                  n220 = Unbundle By Name(w176) -> ("测量值"=w175:sgl, "信号值"=w174:sgl, "温度测量值"=w173:sgl, "数据标识"=w172:string)
                  n221 = Get Date/Time In Seconds() -> (seconds since 1Jan1904=w186:timestamp)
                  n222 = Bundle By Name(cluster=T1 {"时间"=timestamp(0 s since 1904-01-01), "测量模式"="水样测试", "数据类型"="N", "检测值"=0.0, "单位"="mg/L", "数据标识"="N", "信号值"=0.0, "标样参考值"=0.0, "因子编码"="", "探头温度"=0.0, "LastTime"=timestamp(0 s since 1904-01-01)} ("data"), "时间"=w186, "测量模式"="水样测试", "数据类型"=w184, "检测值"=w175, "单位"="mg/L", "数据标识"="N" ("水样数据标识"), "信号值"=w174, "因子编码"="", "探头温度"=w173, "数据标识"=w172) -> (w178:T1)
                  n223 = call "data insert.vi"("集成干预"=TRUE, "data"=w178, "table in"="氨氮") -> ("error out"=w180:errorcluster)  [unwired: 8 in]
                  n224 = Unbundle By Name(w180) -> ("status"=w181:bool)
                  n225 = Not(x=w181) -> (.not. x?=w188:bool)
                }
              }
            }
            n226 = case shown="True" w105 {
              tunnel: w75 -> [_ w390]
              tunnel: w98 -> [_ w388]
              frame False {
              }
              frame True {
                n227 = global read "多参数全局变量.vi" "盐度显示"() -> (w387:T4)
                n228 = for {
                  N: 10 -> [_]
                  tunnel: w390 -> [w398]
                  tunnel: w388 -> [w410]
                  tunnel: w387 -> [w397]
                  stop <- w415 stop-if-true
                  n229 = Unbundle By Name(w397) -> ("测量值"=w399:sgl, "温度测量值"=w400:sgl, "信号值"=w403:sgl, "数据标识"=w406:string)
                  n230 = Unbundle By Name(w410) -> ("测量值"=w419:sgl, "温度测量值"=w418:sgl, "信号值"=w413:sgl, "数据标识"=w409:string)
                  n231 = Get Date/Time In Seconds() -> (seconds since 1Jan1904=w402:timestamp)
                  n232 = Get Date/Time In Seconds() -> (seconds since 1Jan1904=w414:timestamp)
                  n233 = Bundle By Name(cluster=T1 {"时间"=timestamp(0 s since 1904-01-01), "测量模式"="水样测试", "数据类型"="N", "检测值"=0.0, "单位"="mg/L", "数据标识"="N", "信号值"=0.0, "标样参考值"=0.0, "因子编码"="", "探头温度"=0.0, "LastTime"=timestamp(0 s since 1904-01-01)} ("data"), "因子编码"="", "单位"="ppt", "时间"=w402, "检测值"=w399, "探头温度"=w400, "信号值"=w403, "测量模式"="水样测试", "数据类型"=w398, "数据标识"=w406) -> (w405:T1)
                  n234 = Bundle By Name(cluster=T1 {"时间"=timestamp(0 s since 1904-01-01), "测量模式"="水样测试", "数据类型"="N", "检测值"=0.0, "单位"="mg/L", "数据标识"="N", "信号值"=0.0, "标样参考值"=0.0, "因子编码"="", "探头温度"=0.0, "LastTime"=timestamp(0 s since 1904-01-01)} ("data"), "因子编码"="电导率", "单位"="μS/cm", "时间"=w414, "检测值"=w419, "探头温度"=w418, "信号值"=w413, "测量模式"="水样测试", "数据类型"=w398, "数据标识"=w409) -> (w411:T1)
                  n235 = call "data insert.vi"("集成干预"=TRUE, "data"=w411, "table in"="电导率" ("table输入")) -> ("error out"=w394:errorcluster)  [unwired: 8 in]
                  n236 = call "data insert.vi"("error in (no error)"=w394, "集成干预"=TRUE, "data"=w405, "table in"="盐度") -> ("error out"=w393:errorcluster)  [unwired: 7 in]
                  n237 = Unbundle By Name(w393) -> ("status"=w417:bool)
                  n238 = Not(x=w417) -> (.not. x?=w415:bool)
                }
              }
            }
          }
        }
      }
      frame "结束" {
        w485 = u16 0 items=["空闲", "水样测试", "标样核查"] ("多参数运行状态")
        n239 = case shown="True" w481 {
          frame False {
          }
          frame True {
            n240 = call "操作日志.vi"("日志信息"="【集成干预】结束") -> ()  [unwired: 10 in, 1 out]
          }
        }
      }
    }
    "运行状态" <- w31
    n241 = Format Into String(format string=w39, w25) -> (resulting string=→"多参数运行日志":string)  [unwired: 2 in, 1 out]
    n242 = global write "多参数全局变量.vi" "多参数运行状态"(w31) -> ()
  }
